vi "Unreplace Characters.vi"(0 "String In":string) -> (2 "String Out":string)   [LabVIEW 2015]
doc: "This VI was created for use with the Read/Write Cluster VIs. It converts any carriage return or line feed unique identifier strings in the string to carriage return and line feed characters.\n\nFreeware from Moore Good Ideas, www.mooregoodideas.com. Do not remove this line."
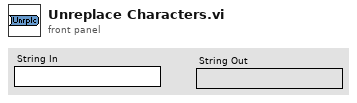
[diagram p1: front panel]
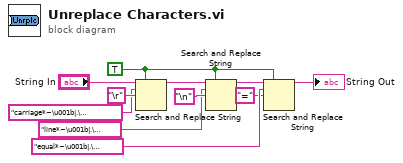
[diagram p0: block diagram]
diagram:
  w3 = TRUE ("replace all? (F)")
  n1 = Search and Replace String(replace all?=w3, input string="String In", search string="carriage*~\u001b|.\u0017return", replace string="\r" ("replace string (\"\")")) -> (result string=w9:string)  [unwired: 1 in, 6 out]
  n2 = Search and Replace String(replace all?=w3, input string=w9, search string="line*~\u001b|.\u0017feed", replace string="\n" ("replace string (\"\")")) -> (result string=w5:string)  [unwired: 1 in, 6 out]
  n3 = Search and Replace String(replace all?=w3, input string=w5, search string="equal*~\u001b|.\u0017sign", replace string="=" ("replace string (\"\")")) -> (result string=→"String Out":string)  [unwired: 1 in, 6 out]
